vi "Mecanum Drive.vi"(8 "Channels":string[](array[string]), 9 "Enum":T2, 11 "Motor Power":T1) -> ()   [LabVIEW 2014]
uses:
  TypeDefs/SRE Enum.ctl
  <vilib>/Rock Robotics/WPI/MotorControl/WPI_MotorControlOpen Talon.vi
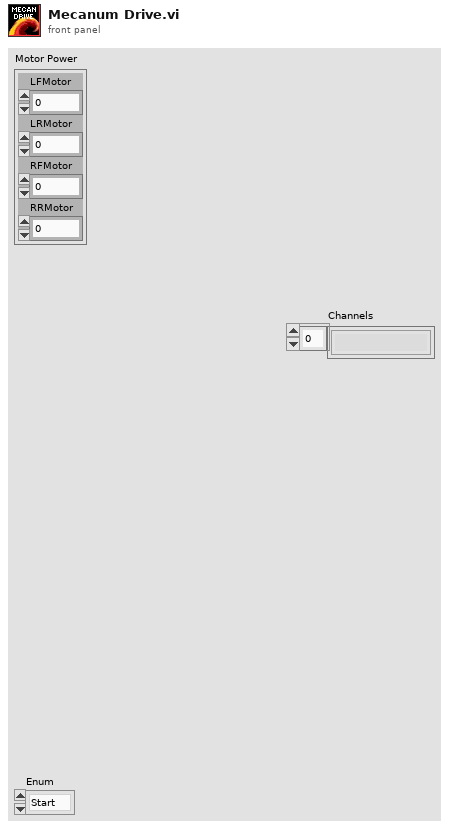
[diagram p1: front panel]
types:
  T1 = cluster{"LFMotor":dbl, "LRMotor":dbl, "RFMotor":dbl, "RRMotor":dbl}
  T2 = typedef "SRE Enum.ctl" = enum16{"Start", "Run", "End"}
  T3 = typedef "WPI_MotorControlDeviceRef.ctl" = cluster{"DeviceStatus":errorcluster, "Type":T4, "PWM":cluster{"Controller":T5, "PWM Channel":T6, "DeadBand":T7}, "CAN":cluster{"Device Number":u8, "Control Mode":T8, "Semaphore":T9, "Max Vout":dbl, "TalonSRX Control Mode":T10}, "Invert":bool, "TransformRef":T11, "InvTransformRef":T11}
  T4 = typedef "WPI_MotorControlType.ctl" = enum16{"PWM", "CAN", "CANTalonSRX"}
  T5 = typedef "FPGA_TypedefDigitalModule.ctl" = enum16{"Controller 1"}
  T6 = typedef "FPGA_DIOPWMChannel.ctl" = enum8{"PWM 0", "PWM 1", "PWM 2", "PWM 3", "PWM 4", "PWM 5", "PWM 6", "PWM 7", "PWM 8", "PWM 9", "PWM MXP 0", "PWM MXP 1", "PWM MXP 2", "PWM MXP 3", "PWM MXP 4", "PWM MXP 5", "PWM MXP 6", "PWM MXP 7", "PWM MXP 8", "PWM MXP 9", "Invalid"}
  T7 = typedef "WPI_PWMDeadband.ctl" = cluster{"Name":string, "maxPositivePwm":i32, "minPositivePwm":i32, "centerPwm":i32, "maxNegativePwm":i32, "minNegativePwm":i32, "angularRange":u16}
  T8 = typedef "WPI_CANJaguar_ControlMode.ctl" = enum8{"Percent VBus", "Current", "Speed", "Position", "Voltage"}
  T9 = typedef "Semaphore RefNum" = refnum<k1>
  T10 = typedef "WPI_CANTalonSRX_APIControlMode.ctl" = enum8{"Percent VBus", "Speed", "Position", "Slave", "Unchanged / Invalid"}
  T11 = typedef "WPI_PWMTransform_ConPane.ctl" = refnum<vi>
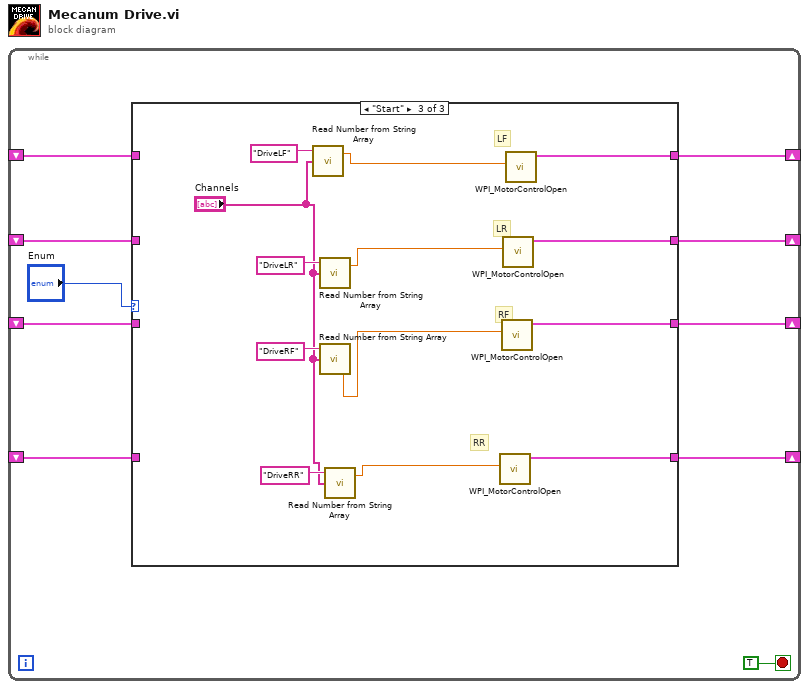
[diagram p0: block diagram]
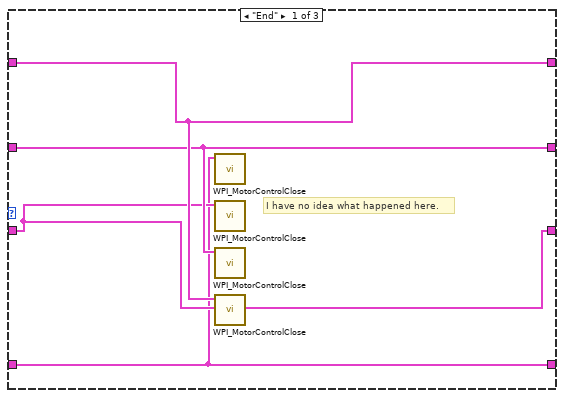
[diagram p2: hidden frame]
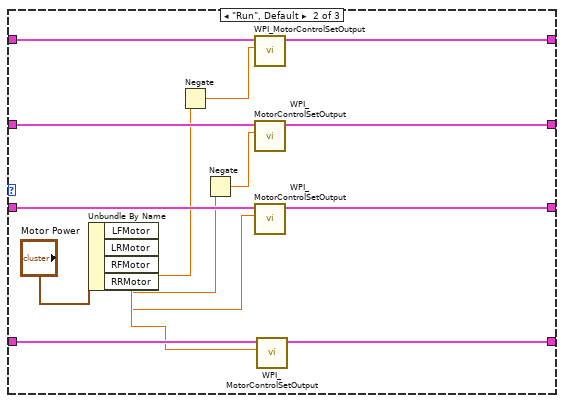
[diagram p3: hidden frame]
diagram:
  n1 = while {
    shift-right: [w9] -> _
    shift-left: _ -> [w2]
    shift-right: [w8] -> _
    shift-left: _ -> [w3]
    shift-right: [w7] -> _
    shift-left: _ -> [w4]
    shift-right: [w6] -> _
    shift-left: _ -> [w5]
    stop <- TRUE stop-if-true
    n2 = case shown="\"Start\"" "Enum" {
      tunnel: [w14 w26 w42] -> w9
      tunnel: [w13 w22 w41] -> w8
      tunnel: [w12 w25 w40] -> w7
      tunnel: [w11 w28 w39] -> w6
      tunnel: w5 -> [w11 w29 _]
      tunnel: w4 -> [w12 w24 _]
      tunnel: w3 -> [w13 w23 _]
      tunnel: w2 -> [w14 w27 _]
      frame "End" {
        # "I have no idea what happened here."
        n3 = call <vilib>:"WPI_MotorControlClose.vi"("MotorControlDevRef"=w11) -> ()  [unwired: 10 in, 1 out]
        n4 = call <vilib>:"WPI_MotorControlClose.vi"("MotorControlDevRef"=w12) -> ()  [unwired: 10 in, 1 out]
        n5 = call <vilib>:"WPI_MotorControlClose.vi"("MotorControlDevRef"=w13) -> ()  [unwired: 10 in, 1 out]
        n6 = call <vilib>:"WPI_MotorControlClose.vi"("MotorControlDevRef"=w14) -> ()  [unwired: 10 in, 1 out]
      }
      frame "Run", Default {
        n7 = Unbundle By Name("Motor Power") -> ("LFMotor"=w18:dbl, "LRMotor"=w19:dbl, "RFMotor"=w20:dbl, "RRMotor"=w21:dbl)
        n8 = Negate(x=w18) -> (-x=w17:dbl)
        n9 = Negate(x=w19) -> (-x=w16:dbl)
        n10 = call <vilib>:"WPI_MotorControlSetOutput.vi"("Output"=w17, "MotorControlDevRef"=w27) -> ("MotorControlDevRef"=w26:T3)  [unwired: 7 in, 2 out]
        n11 = call <vilib>:"WPI_MotorControlSetOutput.vi"("Output"=w16, "MotorControlDevRef"=w23) -> ("MotorControlDevRef"=w22:T3)  [unwired: 7 in, 2 out]
        n12 = call <vilib>:"WPI_MotorControlSetOutput.vi"("Output"=w20, "MotorControlDevRef"=w24) -> ("MotorControlDevRef"=w25:T3)  [unwired: 7 in, 2 out]
        n13 = call <vilib>:"WPI_MotorControlSetOutput.vi"("Output"=w21, "MotorControlDevRef"=w29) -> ("MotorControlDevRef"=w28:T3)  [unwired: 7 in, 2 out]
      }
      frame "Start" {
        # "RR"
        # "RF"
        # "LR"
        # "LF"
        n14 = call "Read Number from String Array.vi"("Variables"="Channels", "Name"="DriveLF") -> ("number"=w34:dbl)  [unwired: 1 in, 1 out]
        n15 = call "Read Number from String Array.vi"("Variables"="Channels", "Name"="DriveLR") -> ("number"=w32:dbl)  [unwired: 1 in, 1 out]
        n16 = call "Read Number from String Array.vi"("Variables"="Channels", "Name"="DriveRF") -> ("number"=w33:dbl)  [unwired: 1 in, 1 out]
        n17 = call "Read Number from String Array.vi"("Variables"="Channels", "Name"="DriveRR") -> ("number"=w30:dbl)  [unwired: 1 in, 1 out]
        n18 = call-poly <vilib>:"WPI_MotorControlOpen.vi"("PWM Channel"=w30) -> ("MotorControlDeviceRef"=w39:T3)  [unwired: 9 in, 1 out]
        n19 = call-poly <vilib>:"WPI_MotorControlOpen.vi"("PWM Channel"=w33) -> ("MotorControlDeviceRef"=w40:T3)  [unwired: 9 in, 1 out]
        n20 = call-poly <vilib>:"WPI_MotorControlOpen.vi"("PWM Channel"=w32) -> ("MotorControlDeviceRef"=w41:T3)  [unwired: 9 in, 1 out]
        n21 = call-poly <vilib>:"WPI_MotorControlOpen.vi"("PWM Channel"=w34) -> ("MotorControlDeviceRef"=w42:T3)  [unwired: 9 in, 1 out]
      }
    }
  }
